vi "Find Settled Current.vi"(0 "VISA Resource In":refnum<visa-resource-name>, 1 "Channel 1 (Main)":T1, 2 "Measure Function Ch 1":T2, 3 "Channel 2":T1=enum."Channel B", 4 "Measure Function Ch 2":T2, 5 "error in":errorcluster, 6 "Measuring Equipment":enum16{"Source Meter", "Multimeter"}(ring), 7 "Range":dbl=2e-08, 8 "Source Meter Type":enum16{"Single Channel", "Dual Channel"}(ring)) -> (14 "Settled":bool, 15 "Settled Value Ch 1 (Main)":dbl, 16 "Settled Value Ch 2":dbl, 19 "error out":errorcluster)   [LabVIEW 2016]
uses:
  <userlib>/_TI-LA/Instr Drivers/Sourcemeter/Ke 26xx/Driver/EasyIO/Typedefs/Ke 26xx Channel Selection.ctl
  <userlib>/_TI-LA/Instr Drivers/Sourcemeter/Ke 26xx/Driver/EasyIO/Typedefs/Ke 26xx Measure Function.ctl
  <userlib>/_TI-LA/Instr Drivers/Sourcemeter/Ke 26xx/Driver/Ke 26xx.lvlib
panel:
  in  "Tab Control":enum32{"Souce Meter Settings"}(tab)
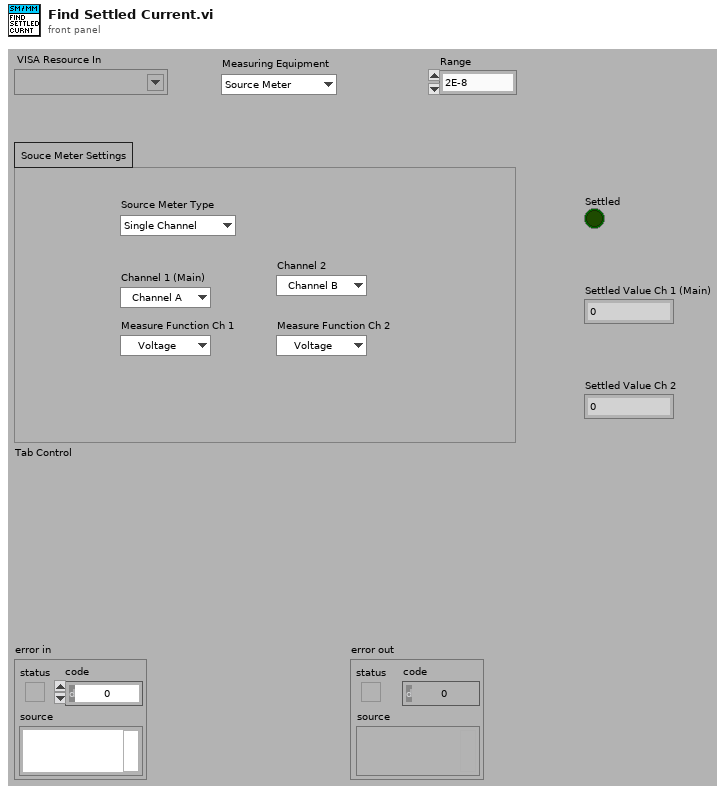
[diagram p1: front panel]
types:
  T1 = typedef "Ke 26xx.lvlib/Ke 26xx Channel Selection.ctl" = enum16{"Channel A", "Channel B"}
  T2 = typedef "Ke 26xx.lvlib/Ke 26xx Measure Function.ctl" = enum16{"Voltage", "Current", "V and I", "Resistance", "Power"}
  T3 = typedef "Ke 26xx.lvlib/Ke 26xx Measurement Data.ctl" = cluster{"Function":T2, "Value 1":dbl, "Value 2":dbl, "Unit 1":T4, "Unit 2":T4}
  T4 = typedef "Ke 26xx.lvlib/Ke 26xx Measurement Unit.ctl" = enum16{"", "V", "A", "Ohms", "W"}
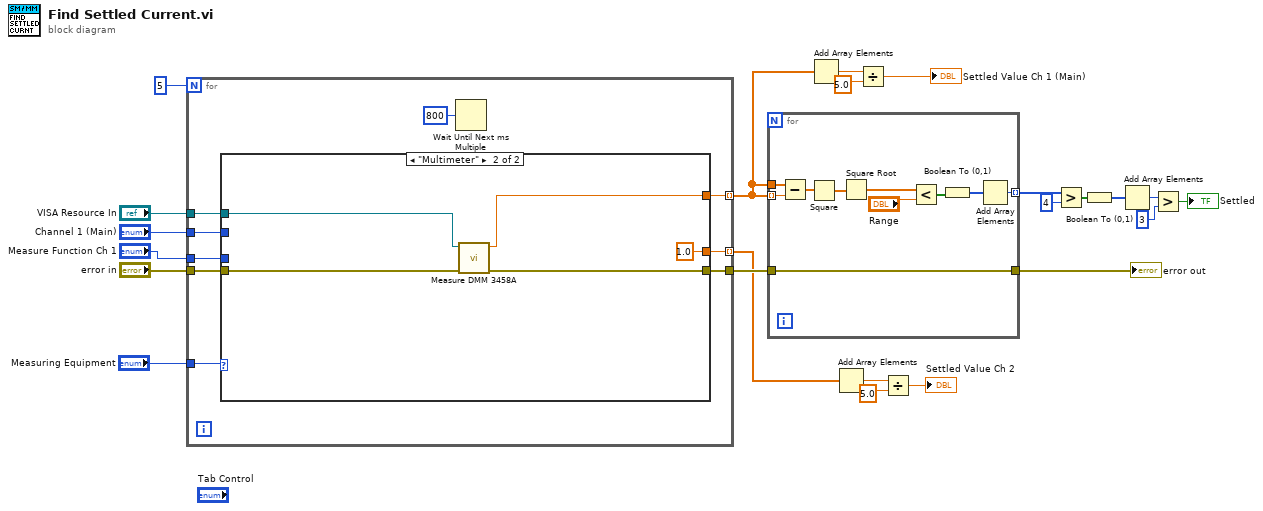
[diagram p0: block diagram]
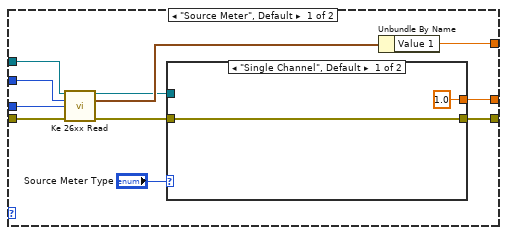
[diagram p2: hidden frame]
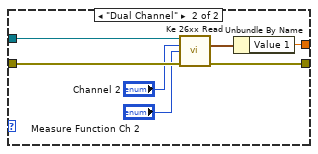
[diagram p3: hidden frame]
diagram:
  n1 = for {
    N: 5 -> [_]
    tunnel: "VISA Resource In" -> [w32]
    tunnel: "Channel 1 (Main)" -> [w26]
    tunnel: "Measure Function Ch 1" -> [w27]
    tunnel: "error in" -> [w31]
    tunnel: [w29] -> w15 mode=indexing
    tunnel: [w28] -> w18
    tunnel: [w25] -> w9 mode=indexing
    tunnel: "Measuring Equipment" -> [w24]
    n2 = case shown="\"Multimeter\"" w24 {
      tunnel: w32 -> [w43 w53]
      tunnel: w31 -> [w42 w56]
      tunnel: [w40 w54] -> w29
      tunnel: [w38 w55] -> w28
      tunnel: w27 -> [w37 _]
      tunnel: w26 -> [w36 _]
      tunnel: [w34 1.0 ("Value 1")] -> w25
      frame "Source Meter", Default {
        n3 = call <userlib>:"Ke 26xx Read.vi"("VISA Resource In"=w43, "Channel"=w36, "Measure Function"=w37, "error in"=w42) -> ("VISA Resource Out"=w35:refnum<visa-resource-name>, "Measured Data"=w41:T3, "error out"=w39:errorcluster)  [unwired: 9 in]
        n4 = case shown="\"Single Channel\", Default" "Source Meter Type" {
          tunnel: w39 -> [w45 w52]
          tunnel: [w45 w51] -> w38
          tunnel: w35 -> [_ w50]
          tunnel: [1.0 ("Value 1") w47] -> w34
          frame "Single Channel", Default {
          }
          frame "Dual Channel" {
            n5 = call <userlib>:"Ke 26xx Read.vi"("VISA Resource In"=w50, "Channel"="Channel 2", "Measure Function"="Measure Function Ch 2", "error in"=w52) -> ("Measured Data"=w48:T3, "error out"=w51:errorcluster)  [unwired: 9 in, 1 out]
            n6 = Unbundle By Name(w48) -> ("Value 1"=w47:dbl)
          }
        }
        n7 = Unbundle By Name(w41) -> ("Value 1"=w40:dbl)
      }
      frame "Multimeter" {
        n8 = call "Measure DMM 3458A.vi"("error in (no error)"=w56, "VISA resource name"=w53) -> ("error out"=w55:errorcluster, "Display Value"=w54:sgl)  [unwired: 8 in]
      }
    }
    n9 = Wait Until Next ms Multiple(millisecond multiple=u32 800) -> ()  [unwired: 1 out]
  }
  n10 = for {
    tunnel: w18 -> [w65]
    tunnel: w15 -> [w63] mode=indexing
    tunnel: w15 -> [w64]
    tunnel: [w66] -> w7 mode=indexing
    tunnel: [w65] -> w16
    n11 = Subtract(x=w64, y=w63) -> (x-y=w62:dbl[])
    n12 = Square(x=w62) -> (x^2=w61:dbl[])
    n13 = Square Root(x=w61) -> (sqrt(x)=w60:dbl[])
    n14 = Less?(x=w60, y="Range") -> (x < y?=w58:bool[])
    n15 = Boolean To (0,1)(Boolean=w58) -> (0, 1=w67:i16[])
    n16 = Add Array Elements(numeric array=w67) -> (sum=w66:i16)
  }
  "error out" <- w16
  n17 = Add Array Elements(numeric array=w15) -> (sum=w14:dbl)
  n18 = Add Array Elements(numeric array=w9) -> (sum=w10:dbl)
  n19 = Divide(x=w14, y=5.0) -> (x/y=→"Settled Value Ch 1 (Main)":dbl)
  n20 = Divide(x=w10, y=5.0) -> (x/y=→"Settled Value Ch 2":dbl)
  n21 = Greater?(x=w7, y=i16 4) -> (0:w5:bool[])
  n22 = Boolean To (0,1)(Boolean=w5) -> (0, 1=w6:i16[])
  n23 = Add Array Elements(numeric array=w6) -> (sum=w4:i16)
  n24 = Greater?(x=w4, y=i16 3) -> (0:→"Settled":bool)
